vi "模块1功能流程.vi"() -> ()   [LabVIEW 2016]
uses:
  <vilib>/Instr/_visa.llb/VISA Configure Serial Port (Instr).vi
panel:
  out "CH0电压（mv）":i32
  out "CH1电压（mv）":i32
  out "CH2电压（mv）":i32
  out "CH3电压（mv）":i32
  in  "停止":bool
  in  "选择输入读取":enum16{"CH0", "CH1", "CH2", "CH3"}(ring)
  out "DI0":bool
  out "DI1":bool
  out "DI2":bool
  out "DI3":bool
  out "DI4":bool
  out "DI5":bool
  out "DI6":bool
  out "DI7":bool
  in  "DO7":bool
  in  "DO0":bool
  in  "DO1":bool
  in  "DO2":bool
  in  "DO3":bool
  in  "DO4":bool
  in  "DO5":bool
  in  "DO6":bool
  out "CH3":bool
  out "CH2":bool
  out "CH1":bool
  out "CH0":bool
  out "CH3电压（mv）":string
  out "CH2电压（mv）":string
  out "CH1电压（mv）":string
  out "CH0电压（mv）":string
  # "数字变送器模块手动调试"
  # "D5131(模拟量输入）"
  # "D1701(数字输入输出）"
  # "数字输出"
  # "数字输入"
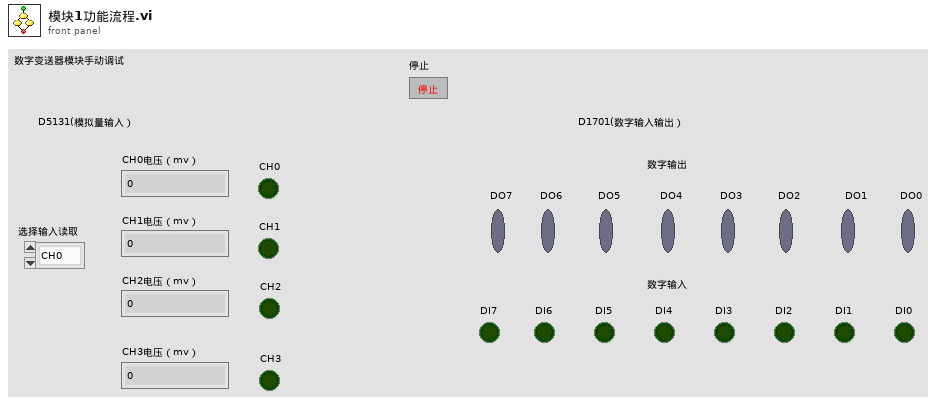
[diagram p1: front panel]
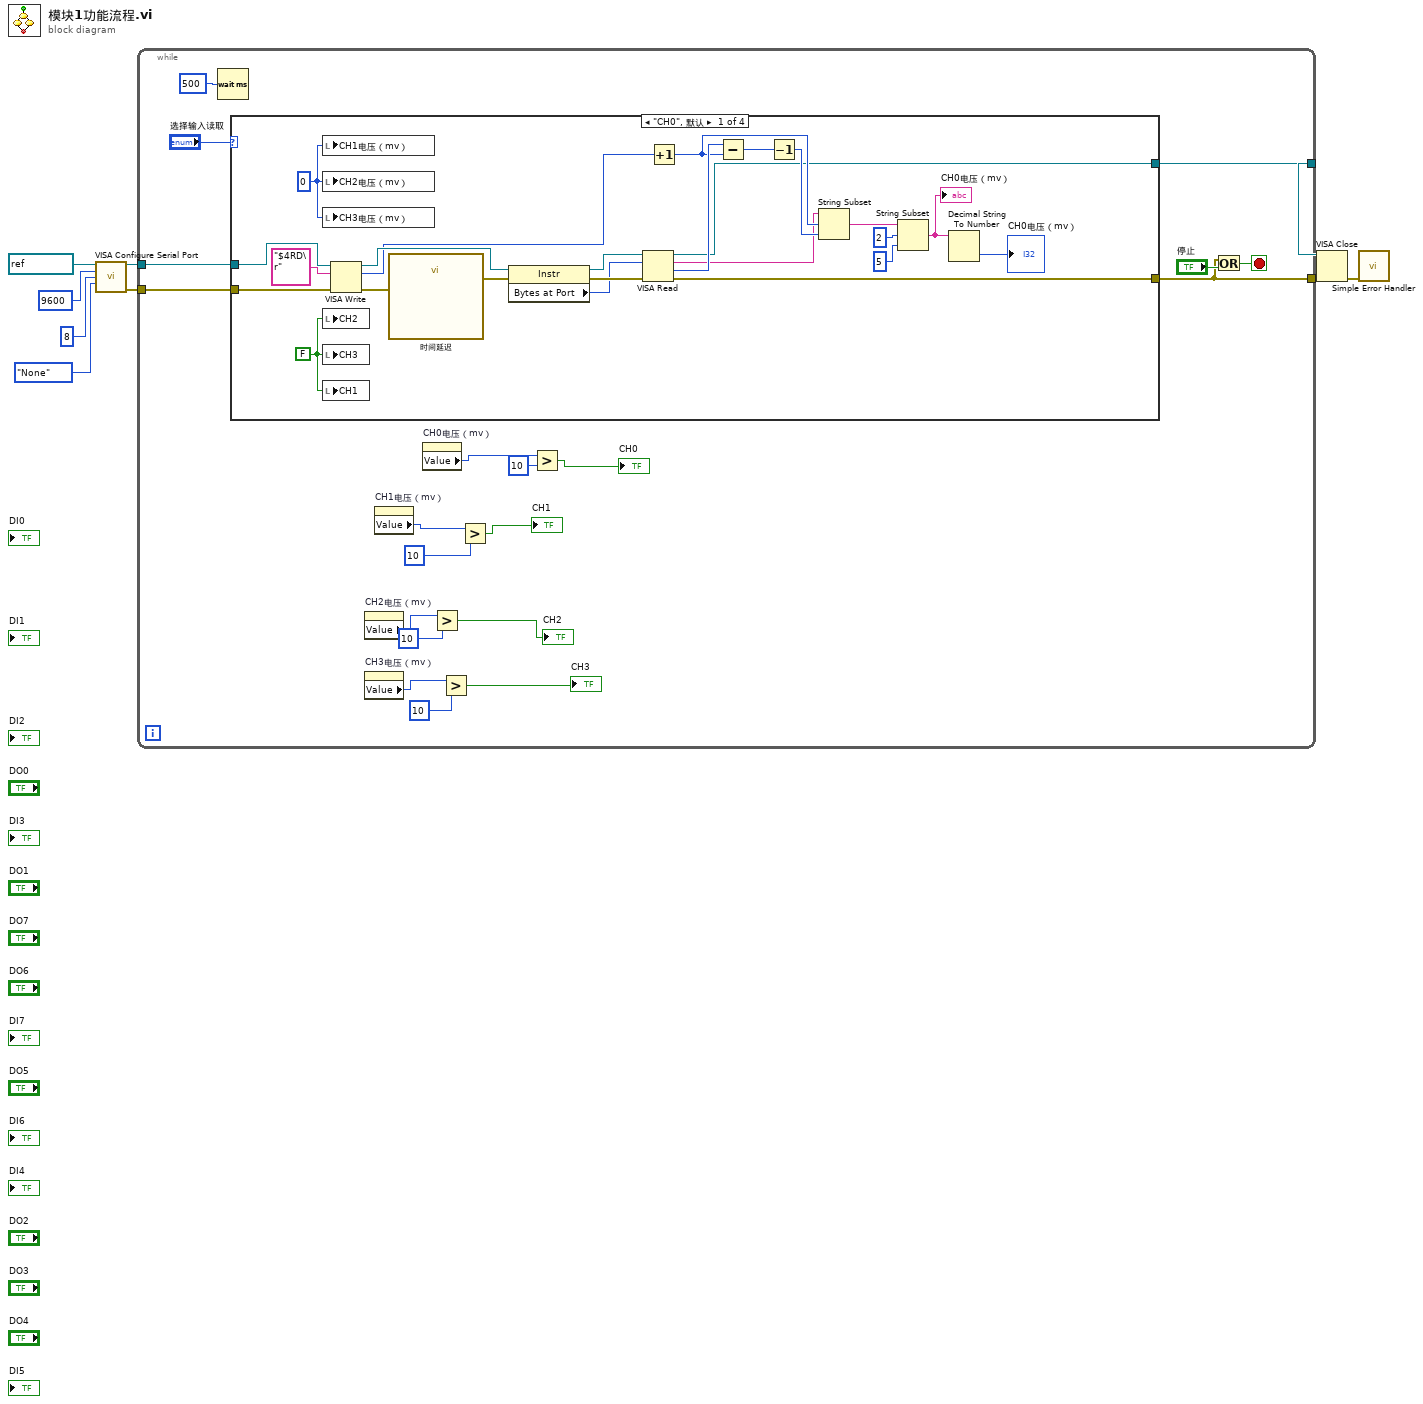
[diagram p0: block diagram]
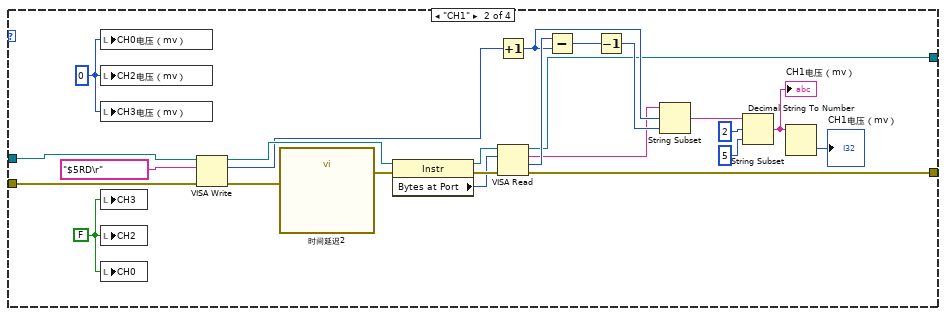
[diagram p2: hidden frame]
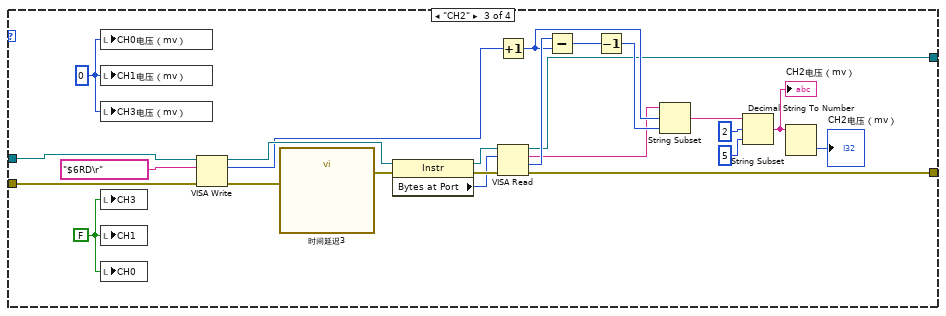
[diagram p3: hidden frame]
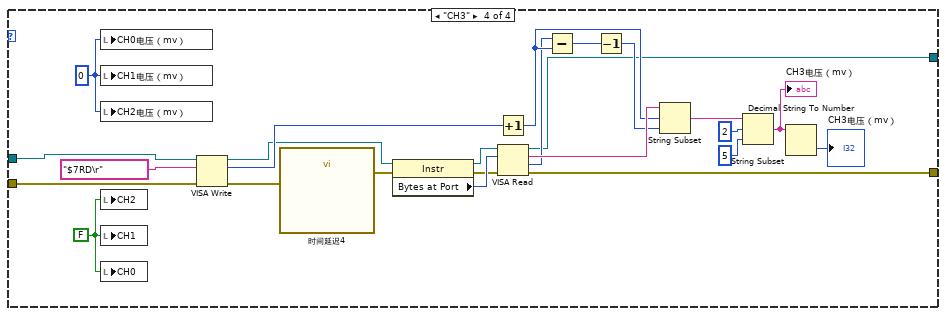
[diagram p4: hidden frame]
diagram:
  n1 = call-poly "VISA Configure Serial Port"("VISA resource name"=refnum<visa-resource-name> "COM3", "baud rate (9600)"=u32 9600, "data bits (8)"=u16 8, "parity (0:none)"=enum16{"None", "Odd", "Even", "Mark", "Space"}."None") -> ("VISA resource name out"=w5:refnum<visa-resource-name>, "error out"=w4:errorcluster)  [unwired: 10 in]
  n2 = while {
    tunnel: w5 -> [w28]
    tunnel: w4 -> [w27]
    tunnel: [w26] -> w3
    tunnel: [w23] -> w2
    stop <- w24 stop-if-true
    n3 = Wait (ms)(milliseconds to wait=u32 500 ("等待时间（毫秒）")) -> ()  [unwired: 1 out]
    n4 = case shown="\"CH0\", 默认" "选择输入读取" {
      tunnel: w28 -> [w53 w64 w88 w112]
      tunnel: w27 -> [w45 w63 w87 w111]
      tunnel: [w38 w62 w86 w110] -> w26
      tunnel: [w37 w61 w85 w109] -> w23
      frame "CH0", Default {
        w30 = 0
        w36 = FALSE
        n5 = local write "CH1电压（mv）"(w30) -> ()
        n6 = local write "CH2电压（mv）"(w30) -> ()
        n7 = local write "CH3电压（mv）"(w30) -> ()
        n8 = local write "CH2"(w36) -> ()
        n9 = local write "CH3"(w36) -> ()
        n10 = local write "CH1"(w36) -> ()
        n11 = VISA Write(VISA resource name=w53, write buffer="$4RD\r", error in (no error)=w45) -> (VISA resource name out=w51:refnum<visa-resource-name>, return count=w44:u32, error out=w46:errorcluster)
        n12 = call "时间延迟"("error in (no error)"=w46) -> ("error out"=w47:errorcluster)  [unwired: 10 in]
        n13 = property class="Instr"(reference=w51, error in=w47) -> (reference out=w48:refnum<visa-resource-name>, error out=w50:errorcluster, "Bytes at Port"=w49:u32)
        n14 = VISA Read(VISA resource name=w48, byte count=w49, error in (no error)=w50) -> (VISA resource name out=w38:refnum<visa-resource-name>, read buffer=w39:string, return count=w43:u32, error out=w37:errorcluster)
        n15 = Increment(x=w44) -> (x+1=w41:u32)
        n16 = Subtract(x=w43, y=w41) -> (x-y=w42:u32)
        n17 = Decrement(x=w42) -> (x-1=w40:u32)
        n18 = String Subset(string=w39, offset (0)=w41, length (rest)=w40) -> (substring=w35:string)
        n19 = String Subset(string=w35, offset (0)=2 ("偏移量(0)"), length (rest)=5 ("长度（剩余）")) -> (substring=w32:string)
        "CH0电压（mv）" <- w32
        n20 = Decimal String To Number(string=w32) -> (number=→"CH0电压（mv）":i32)  [unwired: 2 in, 1 out]
      }
      frame "CH1" {
        w54 = 0
        w60 = FALSE
        n21 = local write "CH0电压（mv）"(w54) -> ()
        n22 = local write "CH2电压（mv）"(w54) -> ()
        n23 = local write "CH3电压（mv）"(w54) -> ()
        n24 = local write "CH3"(w60) -> ()
        n25 = local write "CH2"(w60) -> ()
        n26 = local write "CH0"(w60) -> ()
        n27 = VISA Write(VISA resource name=w64, write buffer="$5RD\r", error in (no error)=w63) -> (VISA resource name out=w76:refnum<visa-resource-name>, return count=w70:u32, error out=w71:errorcluster)
        n28 = call "时间延迟2"("error in (no error)"=w71) -> ("error out"=w72:errorcluster)  [unwired: 10 in]
        n29 = property class="Instr"(reference=w76, error in=w72) -> (reference out=w73:refnum<visa-resource-name>, error out=w75:errorcluster, "Bytes at Port"=w74:u32)
        n30 = Increment(x=w70) -> (x+1=w67:u32)
        n31 = VISA Read(VISA resource name=w73, byte count=w74, error in (no error)=w75) -> (VISA resource name out=w62:refnum<visa-resource-name>, read buffer=w65:string, return count=w69:u32, error out=w61:errorcluster)
        n32 = Subtract(x=w69, y=w67) -> (x-y=w68:u32)
        n33 = Decrement(x=w68) -> (x-1=w66:u32)
        n34 = String Subset(string=w65, offset (0)=w67, length (rest)=w66) -> (substring=w59:string)
        n35 = String Subset(string=w59, offset (0)=2 ("偏移量(0)"), length (rest)=5 ("长度（剩余）")) -> (substring=w56:string)
        "CH1电压（mv）" <- w56
        n36 = Decimal String To Number(string=w56) -> (number=→"CH1电压（mv）":i32)  [unwired: 2 in, 1 out]
      }
      frame "CH2" {
        w78 = 0
        w84 = FALSE
        n37 = local write "CH0电压（mv）"(w78) -> ()
        n38 = local write "CH1电压（mv）"(w78) -> ()
        n39 = local write "CH3电压（mv）"(w78) -> ()
        n40 = local write "CH3"(w84) -> ()
        n41 = local write "CH1"(w84) -> ()
        n42 = local write "CH0"(w84) -> ()
        n43 = VISA Write(VISA resource name=w88, write buffer="$6RD\r", error in (no error)=w87) -> (VISA resource name out=w100:refnum<visa-resource-name>, return count=w94:u32, error out=w95:errorcluster)
        n44 = call "时间延迟3"("error in (no error)"=w95) -> ("error out"=w96:errorcluster)  [unwired: 10 in]
        n45 = property class="Instr"(reference=w100, error in=w96) -> (reference out=w97:refnum<visa-resource-name>, error out=w99:errorcluster, "Bytes at Port"=w98:u32)
        n46 = Increment(x=w94) -> (x+1=w91:u32)
        n47 = VISA Read(VISA resource name=w97, byte count=w98, error in (no error)=w99) -> (VISA resource name out=w86:refnum<visa-resource-name>, read buffer=w89:string, return count=w93:u32, error out=w85:errorcluster)
        n48 = Subtract(x=w93, y=w91) -> (x-y=w92:u32)
        n49 = Decrement(x=w92) -> (x-1=w90:u32)
        n50 = String Subset(string=w89, offset (0)=w91, length (rest)=w90) -> (substring=w83:string)
        n51 = String Subset(string=w83, offset (0)=2 ("偏移量(0)"), length (rest)=5 ("长度（剩余）")) -> (substring=w80:string)
        "CH2电压（mv）" <- w80
        n52 = Decimal String To Number(string=w80) -> (number=→"CH2电压（mv）":i32)  [unwired: 2 in, 1 out]
      }
      frame "CH3" {
        w102 = 0
        w108 = FALSE
        n53 = local write "CH0电压（mv）"(w102) -> ()
        n54 = local write "CH1电压（mv）"(w102) -> ()
        n55 = local write "CH2电压（mv）"(w102) -> ()
        n56 = local write "CH2"(w108) -> ()
        n57 = local write "CH1"(w108) -> ()
        n58 = local write "CH0"(w108) -> ()
        n59 = VISA Write(VISA resource name=w112, write buffer="$7RD\r", error in (no error)=w111) -> (VISA resource name out=w114:refnum<visa-resource-name>, return count=w120:u32, error out=w119:errorcluster)
        n60 = call "时间延迟4"("error in (no error)"=w119) -> ("error out"=w118:errorcluster)  [unwired: 10 in]
        n61 = property class="Instr"(reference=w114, error in=w118) -> (reference out=w117:refnum<visa-resource-name>, error out=w115:errorcluster, "Bytes at Port"=w116:u32)
        n62 = Increment(x=w120) -> (x+1=w123:u32)
        n63 = VISA Read(VISA resource name=w117, byte count=w116, error in (no error)=w115) -> (VISA resource name out=w110:refnum<visa-resource-name>, read buffer=w125:string, return count=w121:u32, error out=w109:errorcluster)
        n64 = Subtract(x=w121, y=w123) -> (x-y=w122:u32)
        n65 = Decrement(x=w122) -> (x-1=w124:u32)
        n66 = String Subset(string=w125, offset (0)=w123, length (rest)=w124) -> (substring=w107:string)
        n67 = String Subset(string=w107, offset (0)=2 ("偏移量(0)"), length (rest)=5 ("长度（剩余）")) -> (substring=w104:string)
        "CH3电压（mv）" <- w104
        n68 = Decimal String To Number(string=w104) -> (number=→"CH3电压（mv）":i32)  [unwired: 2 in, 1 out]
      }
    }
    n69 = property on="CH2电压（mv）" class="DigNum (严格)"() -> ("Value"=w18:i32)  [unwired: 2 in, 2 out]
    n70 = property on="CH3电压（mv）" class="DigNum (严格)"() -> ("Value"=w21:i32)  [unwired: 2 in, 2 out]
    n71 = property on="CH1电压（mv）" class="DigNum (严格)"() -> ("Value"=w15:i32)  [unwired: 2 in, 2 out]
    n72 = property on="CH0电压（mv）" class="DigNum (严格)"() -> ("Value"=w12:i32)  [unwired: 2 in, 2 out]
    n73 = Greater?(x=w18, y=10) -> (0:→"CH2":bool)
    n74 = Greater?(x=w21, y=10) -> (0:→"CH3":bool)
    n75 = Greater?(x=w15, y=10) -> (0:→"CH1":bool)
    n76 = Greater?(x=w12, y=10) -> (0:→"CH0":bool)
    n77 = Or(x=w23, y="停止") -> (x .or. y?=w24:bool)
  }
  n78 = VISA Close(VISA resource name=w3, error in (no error)=w2) -> (error out=w1:errorcluster)
  n79 = call <vilib>:"Simple Error Handler.vi"("error in (no error)"=w1) -> ()  [unwired: 4 in, 5 out]
